vi "TrapDSamp.vi"(0 "Trap Data":dbl[][](array[numeric]), 1 "Data Period (s)":dbl, 2 "Trap Disp. dSamp":i32, 3 "Time Stamp":timestamp, 4 "Channel Names":string[](array[string])) -> (14 "Trap dSampd":waveform(dbl)[](array[waveform]), 17 "Trap Raw":waveform(dbl)[](array[waveform]))   [LabVIEW 2013]
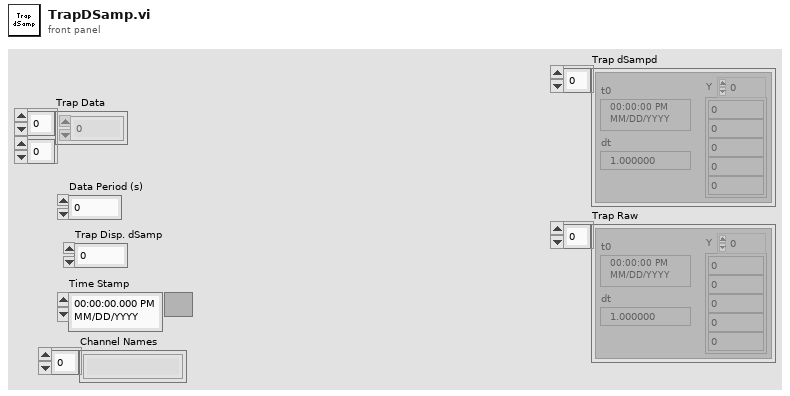
[diagram p1: front panel]
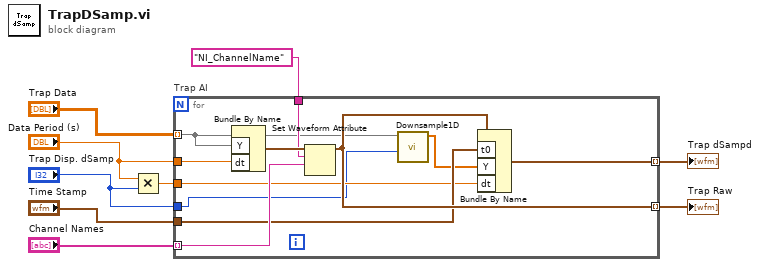
[diagram p0: block diagram]
diagram:
  n1 = Multiply(x="Data Period (s)", y="Trap Disp. dSamp") -> (x*y=w1:dbl)
  n2 = for "Trap AI" {
    tunnel: [w20] -> w5 mode=indexing
    tunnel: "Time Stamp" -> [w14]
    tunnel: "Trap Disp. dSamp" -> [w11]
    tunnel: "Trap Data" -> [w12] mode=indexing
    tunnel: "Data Period (s)" -> [w18]
    tunnel: "Channel Names" -> [w17] mode=indexing
    tunnel: "NI_ChannelName" ("name") -> [w16]
    tunnel: [w15] -> w4 mode=indexing
    tunnel: w1 -> [w13]
    n3 = Bundle By Name("Y"=w12, "dt"=w18) -> (w19:waveform(dbl))  [unwired: 1 out]
    n4 = Set Waveform Attribute(5:w17, 6:w16, 7:w19) -> (3:w15:waveform(dbl))  [unwired: 1 in, 2 out]
    n5 = call "Downsample1D.vi"("Avg N"=w11, "Array In"=w12) -> ("Array Out"=w10:dbl[])  [unwired: 9 in]
    n6 = Bundle By Name(cluster=w15, "t0"=w14, "Y"=w10, "dt"=w13) -> (w20:waveform(dbl))
  }
  "Trap dSampd" <- w5
  "Trap Raw" <- w4
